vi "PixeLink MonitorAndSave_old.vi"(7 "Racine chemin de sauvegarde":path=path "G:/Développement de Programmes/Programmes/octo-labview/PixeLink - Homebrew/Data") -> ()   [LabVIEW 2014]
uses:
  <vilib>/addons/PixeLINK/Low Level Functions/ACQUISITION.llb/TDPU-Acquisition-StreamState.ctl
  <vilib>/addons/PixeLINK/Low Level Functions/CAMERA_FEATURES.llb/TDPU-CameraFeatures-FeatureIds.ctl
  <vilib>/addons/PixeLINK/Low Level Functions/CAMERA_FEATURES.llb/TDPU-CameraFeatures-FeatureFlags.ctl
panel:
  in  "Refresh Exposure":bool
  out "Div":dbl
  out "Imager Serial #":u32[](array[numeric])
  in  "Chemins de sauvegarde":path[](array[path])
  in  "Bind Path to Camera":bool
  in  "Automatic\nfolder naming":bool=TRUE
  in  "Imager":u32(ring)=741003962 items=["Cam 0"=95300230]
  out "Error OUT 2":errorcluster
  out "Error OUT":errorcluster
  in  "Overwrite?":bool
  in  "Snap current Data":bool
  in  "Save Data":bool
  out "Warning":bool
  out "Message":string
  in  "Indice":u32
  in  "Nom du fichier":string="tir"
  in  "Mode de Sauvegarde":u16(ring)=1 items=["Manuel", "Automatique"]
  out "Captured Image":dbl[][](graph)
  out "Waiting for Trigger":bool
  in  "Continuous Grab":bool
  in  "Snap Next frame":bool
  out "Camera Handle":u32
  in  "Stop Grab":bool
  in  "Trigger Type":enum16{"Free Running", "Software", "Hardware"}(ring)
  in  "Trigger Polarity":enum16{"Positive", "Negative"}(ring)
  in  "Refresh Trigger":bool
  in  "Exposure Time":dbl(slide) min=6.350000330712646e-05 max=10.0 scale=6.350000330712646e-05..10.0
  in  "stop":bool
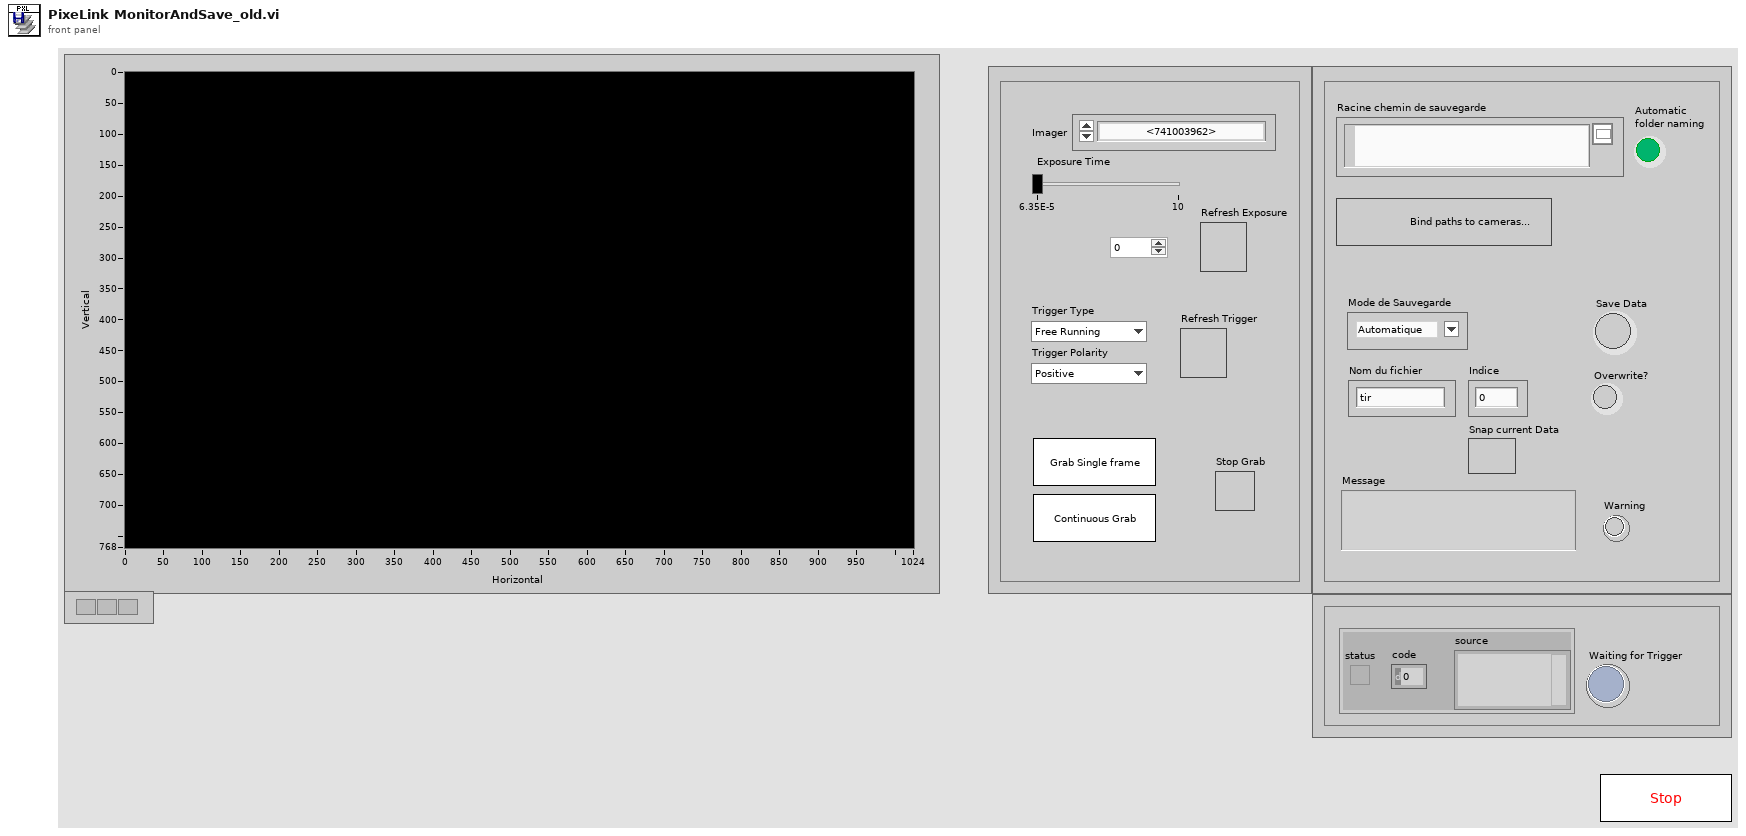
[diagram p1: front panel]
types:
  T1 = typedef "LVStringsAndValuesArrayTypeDef_U32.ctl" = cluster{"String":string, "Value":u32}[]
  T2 = typedef "TDPU-CameraFeatures-FeatureFlags.ctl" = u32
  T3 = typedef "TDPU-CameraFeatures-FeatureIds.ctl" = u32
  T4 = typedef "TDPU-Acquisition-StreamState.ctl" = u32
  T5 = typedef "TDPU-Identification-Camera_Info.ctl" = cluster{"VendorName":string, "ModelName":string, "Description":string, "SerialNumber":string, "FirmwareVersion":string, "FPGAVersion":string, "CameraName":string}
  T6 = typedef "TDPU-Acquisition-Frame_Desc.ctl" = cluster{"uSize":u32, "fFrameTime":dbl, "uFrameNumber":u32, "Brightness":cluster{"fValue":dbl}, "AutoExposure":cluster{"fValue":dbl}, "Sharpness":cluster{"fValue":dbl}, "WhiteBalance":cluster{"fValue":dbl}, "Hue":cluster{"fValue":dbl}, "Saturation":cluster{"fValue":dbl}, "Gamma":cluster{"fValue":dbl}, "Shutter":cluster{"fValue":dbl}, "Gain":cluster{"fValue":dbl}, "Iris":cluster{"fValue":dbl}, "Focus":cluster{"fValue":dbl}, "Temperature":cluster{"fValue":dbl}, "Trigger":cluster{"fMode":dbl, "fType":dbl, "fPolarity":dbl, "fDelay":dbl, "fParameter":dbl}, "Zoom":cluster{"fValue":dbl}, "Pan":cluster{"fValue":dbl}, "Tilt":cluster{"fValue":dbl}, "OpticalFilter":cluster{"fValue":dbl}, "GPIO":cluster{"fMode":dbl[], "fPolarity":dbl[], "fParameter1":dbl[], "fParameter2":dbl[], "fParameter3":dbl[]}, "FrameRate":cluster{"fValue":dbl}, "ROI":cluster{"fLeft":dbl, "fTop":dbl, "fWidth":dbl, "fHeight":dbl}, "Flip":cluster{"fHorizontal":dbl, "fVertical":dbl}, "PixelAddressingValue":cluster{"fValue":dbl}, "PixelFormat":cluster{"fValue":dbl}, "ExtendedShutter":cluster{"fKneePoint":dbl[]}, "AutoROI":cluster{"fLeft":dbl, "fTop":dbl, "fWidth":dbl, "fHeight":dbl}, "WhiteShading":cluster{"fRedGain":dbl, "fGreenGain":dbl, "fBlueGain":dbl}, "Rotate":cluster{"fValue":dbl}, "PixelAddressingMode":cluster{"fValue":dbl}}
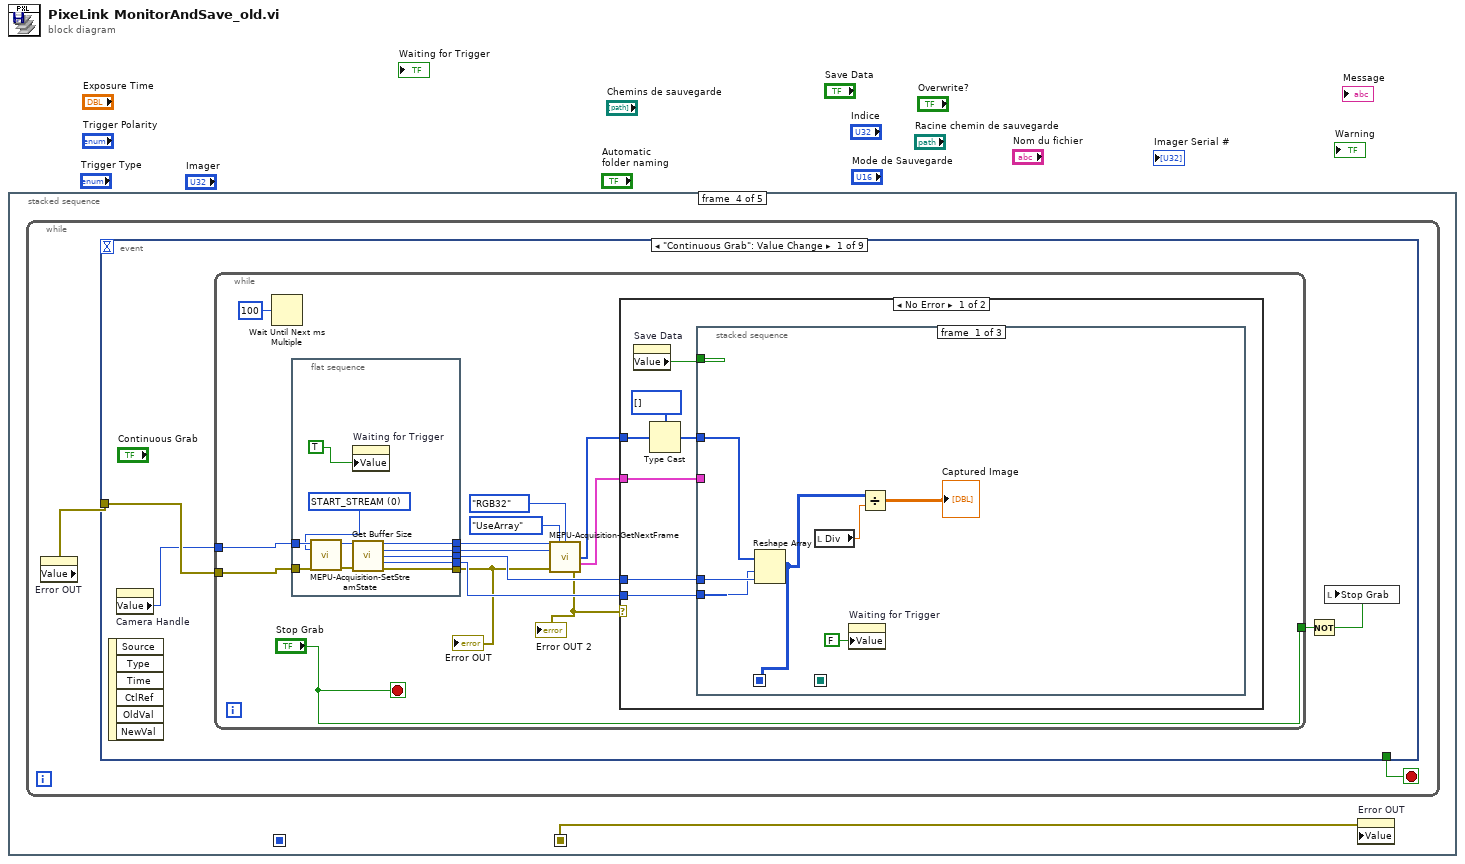
[diagram p0: block diagram]
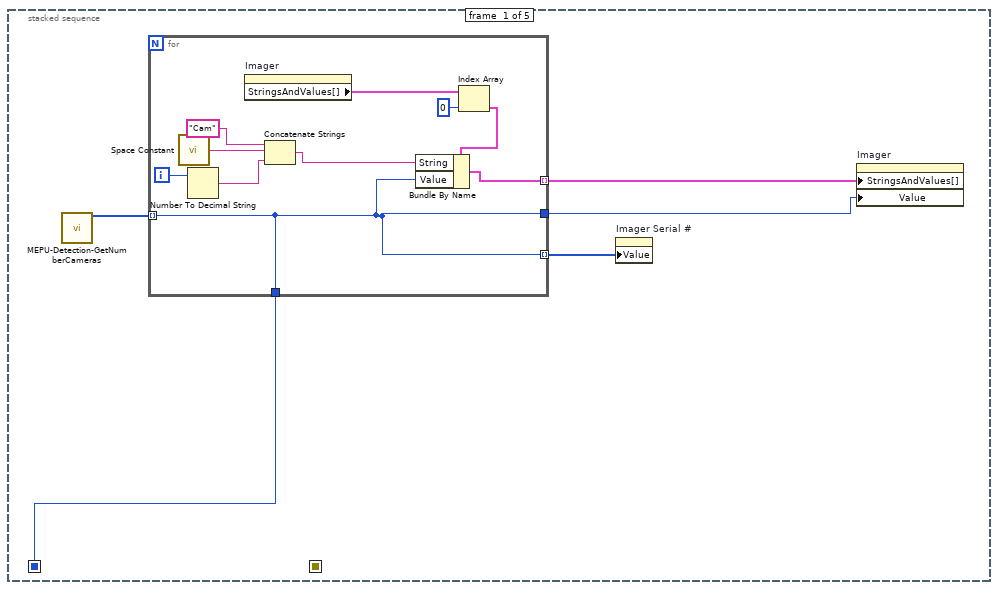
[diagram p2: hidden frame]
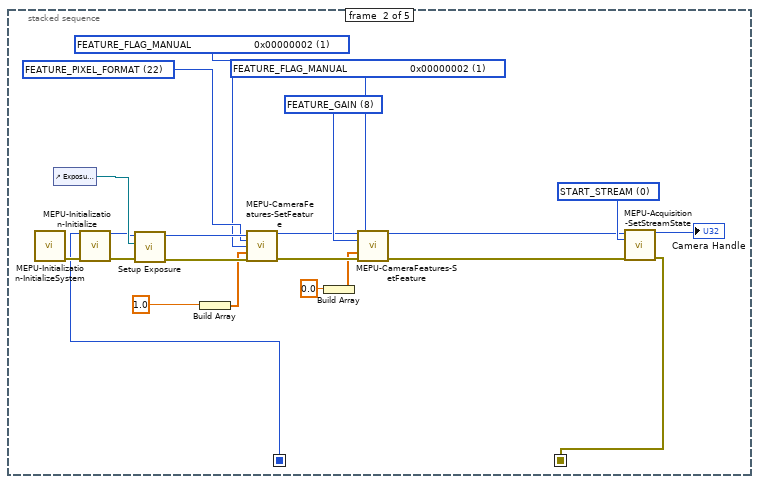
[diagram p3: hidden frame]
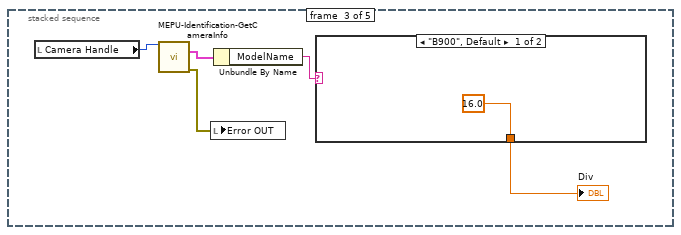
[diagram p4: hidden frame]
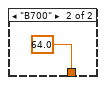
[diagram p5: hidden frame]
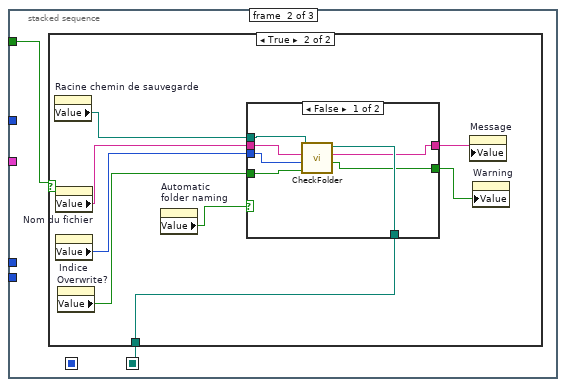
[diagram p6: hidden frame]
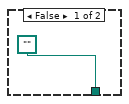
[diagram p7: hidden frame]
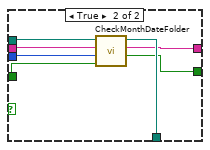
[diagram p8: hidden frame]
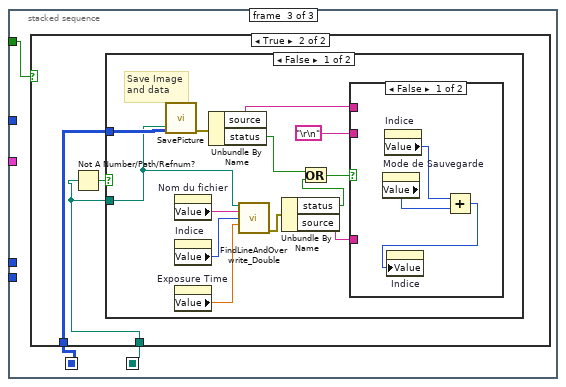
[diagram p9: hidden frame]
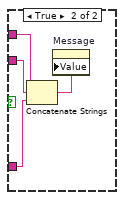
[diagram p11: hidden frame]
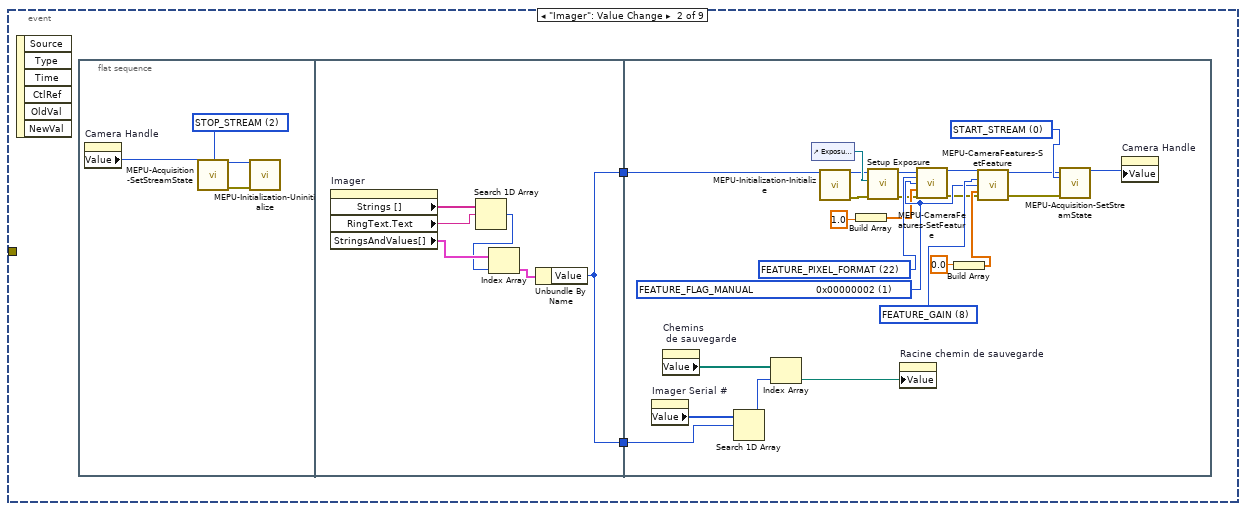
[diagram p14: hidden frame]
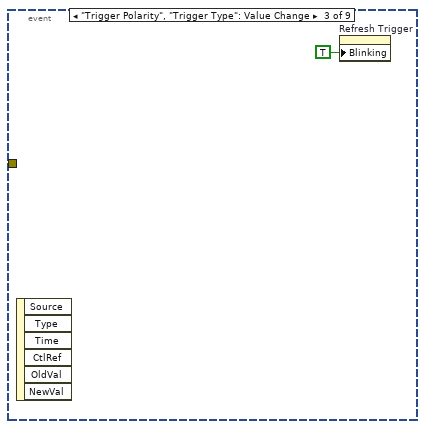
[diagram p15: hidden frame]
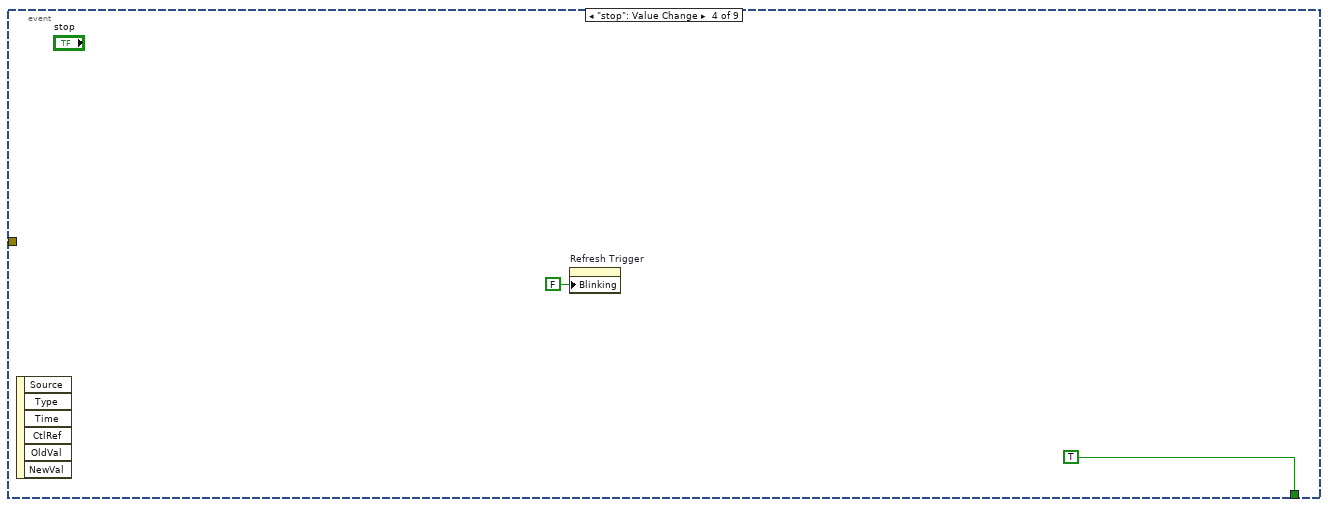
[diagram p16: hidden frame]
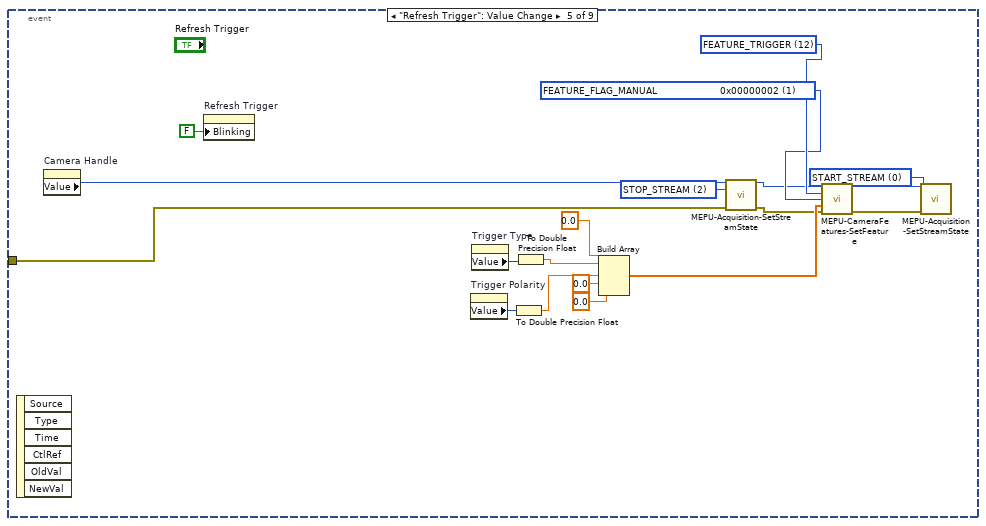
[diagram p17: hidden frame]
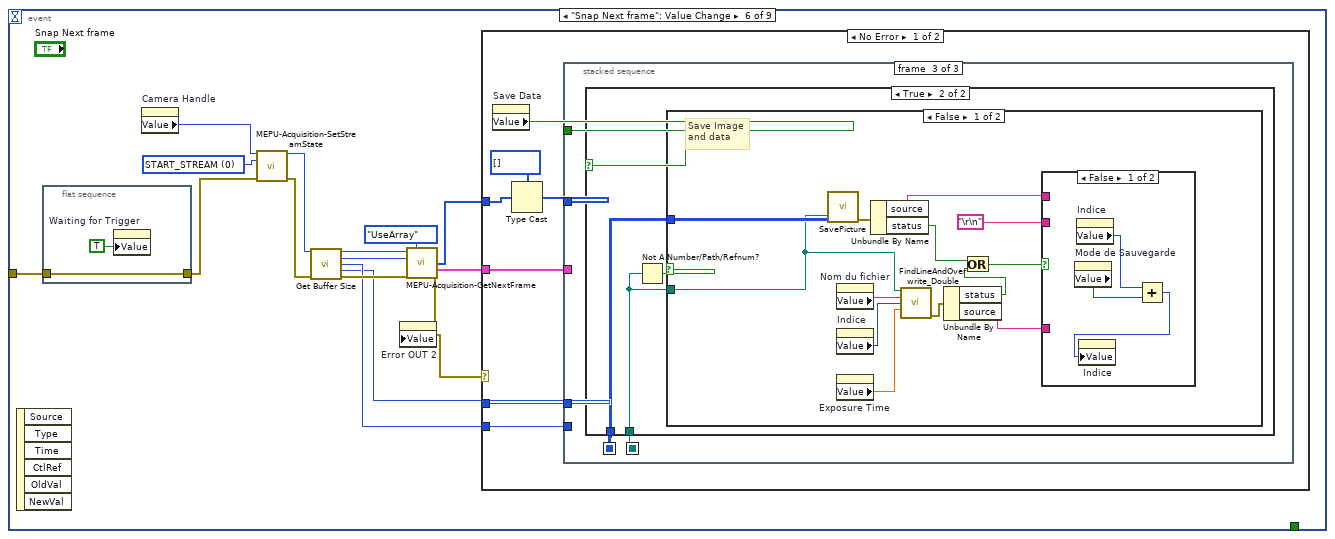
[diagram p18: hidden frame]
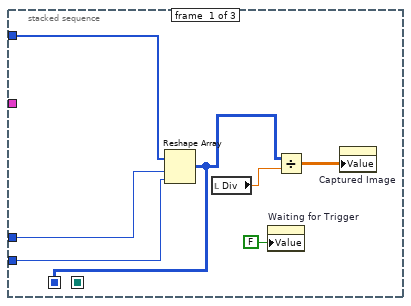
[diagram p19: hidden frame]
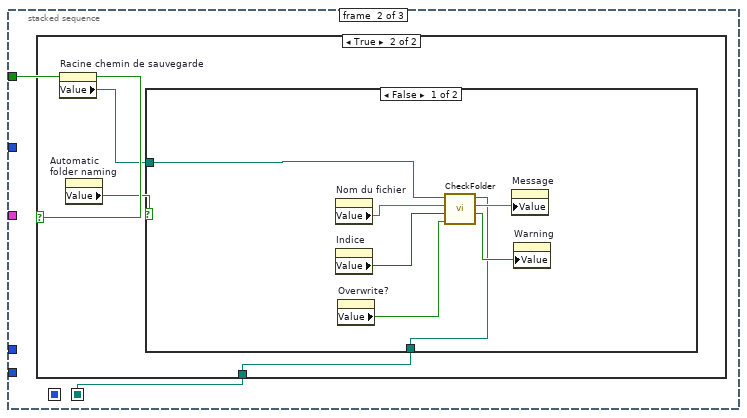
[diagram p20: hidden frame]
diagram:
  n1 = stacked-sequence {
    seq-local: [_ w26 _ _ _] -> [_ _ _ w45 _]
    seq-local: [w4 _ _ _ _] -> [_ w16 _ _ _]
    frame #0 {
      n2 = call <vilib>:"MEPU-Detection-GetNumberCameras.vi"() -> ("LV_SerialNumbers OUT"=w5:u32[])  [unwired: 13 in, 2 out]
      n3 = for {
        tunnel: w5 -> [w6] mode=indexing
        tunnel: [w10] -> w3 mode=indexing
        tunnel: [w6] -> w4
        tunnel: [w6] -> w2
        tunnel: [w6] -> w1 mode=indexing
        i -> [w15]
        n4 = call <vilib>:"Space Constant.vi"() -> ("String"=w13:string)
        n5 = Number To Decimal String(number=w15) -> (decimal integer string=w12:string)  [unwired: 1 in]
        n6 = property on="Imager" class="Ring (strict)"() -> ("StringsAndValues[]"=w9:T1)  [unwired: 2 in, 2 out]
        n7 = Concatenate Strings("Cam", w13, w12) -> (w11:string)
        n8 = Index Array(array=w9, index=0) -> (element=w7:cluster{"String":string, "Value":u32})
        n9 = Bundle By Name(cluster=w7, "String"=w11, "Value"=w6) -> (w10:cluster{"String":string, "Value":u32})
      }
      n10 = property on="Imager Serial #" class="Arr (strict)"("Value"=w1) -> ()  [unwired: 2 in, 2 out]
      n11 = property on="Imager" class="Ring (strict)"("StringsAndValues[]"=w3, "Value"=w2) -> ()  [unwired: 2 in, 2 out]
    }
    frame #1 {
      w21 = T2 1 items=["FEATURE_FLAG_PRESENCE                 0x00000001", "FEATURE_FLAG_MANUAL                     0x00000002", "FEATURE_FLAG_AUTO                         0x00000004", "FEATURE_FLAG_ONEPUSH                   0x00000008", "FEATURE_FLAG_OFF                            0x00000010", "FEATURE_FLAG_DESC_SUPPORTED    0x00000020", "FEATURE_FLAG_READ_ONLY               0x00000040"] ("uFlags IN")
      w20 = T3 8 items=["FEATURE_BRIGHTNESS", "FEATURE_EXPOSURE", "FEATURE_SHARPNESS", "FEATURE_WHITE_BAL", "FEATURE_HUE", "FEATURE_SATURATION", "FEATURE_GAMMA", "FEATURE_SHUTTER", "FEATURE_GAIN", "FEATURE_IRIS", "FEATURE_FOCUS", "FEATURE_TEMPERATURE", "FEATURE_TRIGGER", "FEATURE_ZOOM", "FEATURE_PAN", "FEATURE_TILT", "FEATURE_OPT_FILTER", "FEATURE_GPIO", "FEATURE_FRAME_RATE", "FEATURE_ROI", "FEATURE_FLIP", "FEATURE_PIXEL_ADDRESSING", "FEATURE_PIXEL_FORMAT", "FEATURE_EXTENDED_SHUTTER", "FEATURE_AUTO_ROI", "FEATURE_LOOKUP_TABLE", "FEATURE_MEMORY_CHANNEL", "FEATURE_WHITE_SHADING", "FEATURE_ROTATE", "FEATURE_IMAGER_CLK_DIVISOR", "FEATURE_TRIG_WITH_CNTRLD_LIGHT", "FEATURE_MAX_PIXEL_SIZE"] ("uFeatureId IN")
      w29 = T2 1 items=["FEATURE_FLAG_PRESENCE                 0x00000001", "FEATURE_FLAG_MANUAL                     0x00000002", "FEATURE_FLAG_AUTO                         0x00000004", "FEATURE_FLAG_ONEPUSH                   0x00000008", "FEATURE_FLAG_OFF                            0x00000010", "FEATURE_FLAG_DESC_SUPPORTED    0x00000020", "FEATURE_FLAG_READ_ONLY               0x00000040"] ("uFlags IN")
      w30 = T3 22 items=["FEATURE_BRIGHTNESS", "FEATURE_EXPOSURE", "FEATURE_SHARPNESS", "FEATURE_WHITE_BAL", "FEATURE_HUE", "FEATURE_SATURATION", "FEATURE_GAMMA", "FEATURE_SHUTTER", "FEATURE_GAIN", "FEATURE_IRIS", "FEATURE_FOCUS", "FEATURE_TEMPERATURE", "FEATURE_TRIGGER", "FEATURE_ZOOM", "FEATURE_PAN", "FEATURE_TILT", "FEATURE_OPT_FILTER", "FEATURE_GPIO", "FEATURE_FRAME_RATE", "FEATURE_ROI", "FEATURE_FLIP", "FEATURE_PIXEL_ADDRESSING", "FEATURE_PIXEL_FORMAT", "FEATURE_EXTENDED_SHUTTER", "FEATURE_AUTO_ROI", "FEATURE_LOOKUP_TABLE", "FEATURE_MEMORY_CHANNEL", "FEATURE_WHITE_SHADING", "FEATURE_ROTATE", "FEATURE_IMAGER_CLK_DIVISOR", "FEATURE_TRIG_WITH_CNTRLD_LIGHT", "FEATURE_MAX_PIXEL_SIZE"] ("uFeatureId IN")
      w36 = T4 0 items=["START_STREAM", "PAUSE_STREAM", "STOP_STREAM"] ("uStreamState IN")
      n12 = call <vilib>:"MEPU-Initialization-InitializeSystem.vi"() -> ("Error OUT"=w37:errorcluster)  [unwired: 15 in]
      n13 = control-ref of="Exposure Time"() -> (w35:refnum<vi>)
      n14 = call <vilib>:"MEPU-Initialization-Initialize.vi"("uSerialNumber IN"=w16, "Error IN"=w37) -> ("phCamera OUT"=w34:u32, "Error OUT"=w33:errorcluster)  [unwired: 11 in, 1 out]
      n15 = call "Setup Exposure.vi"("Error IN"=w33, "Shutter"=w35, "hCamera IN"=w34) -> ("Error OUT"=w32:errorcluster, "phCamera OUT"=w31:u32)  [unwired: 7 in]
      n16 = Build Array(1.0) -> (w27:dbl[])
      n17 = call <vilib>:"MEPU-CameraFeatures-SetFeature.vi"("hCamera IN"=w31, "uFeatureId IN"=w30, "uFlags IN"=w29, "pParms IN"=w27, "Error IN"=w32) -> ("hCamera OUT"=w19:u32, "Error OUT"=w24:errorcluster)  [unwired: 8 in, 1 out]
      n18 = Build Array(0.0) -> (w22:dbl[])
      n19 = call <vilib>:"MEPU-CameraFeatures-SetFeature.vi"("hCamera IN"=w19, "uFeatureId IN"=w20, "uFlags IN"=w21, "pParms IN"=w22, "Error IN"=w24) -> ("hCamera OUT"=w18:u32, "Error OUT"=w17:errorcluster)  [unwired: 8 in, 1 out]
      n20 = call <vilib>:"MEPU-Acquisition-SetStreamState.vi"("hCamera IN"=w18, "uStreamState IN"=w36, "Error IN"=w17) -> ("hCamera OUT"=→"Camera Handle":u32, "Error OUT"=w26:errorcluster)  [unwired: 11 in]
    }
    frame #2 {
      n21 = local read "Camera Handle"() -> (w42:u32)
      n22 = call <vilib>:"MEPU-Identification-GetCameraInfo.vi"("hCamera IN"=w42) -> ("pLVCameraInfo OUT"=w41:T5, "Error OUT"=w38:errorcluster)  [unwired: 12 in, 1 out]
      n23 = local write "Error OUT"(w38) -> ()
      n24 = Unbundle By Name(w41) -> ("ModelName"=w40:string)
      n25 = case shown="\"B900\", Default" w40 {
        tunnel: [16.0 64.0] -> w39
        frame "B900", Default {
        }
        frame "B700" {
        }
      }
      "Div" <- w39
    }
    frame #3 {
      n26 = while {
        stop <- w47 stop-if-true
        n27 = property on="Error OUT" class="Clust (strict)"() -> ("Value"=w46:errorcluster)  [unwired: 2 in, 2 out]
        n28 = event shown="[0] \"Continuous Grab\": Value Change" {
          selector: _ -> [_ _ _ _ _ _ _ _ _]
          dyn-events: _ -> [_ _ _ _ _ _ _ _ _]
          timeout: _ -> [_ _ _ _ _ _ _ _ _]
          tunnel: w46 -> [w51 _ _ _ w189 w207 _ _ _]
          tunnel: [_ _ _ TRUE _ _ _ _ _] -> w47
          event "Continuous Grab": Value Change {
            n29 = event-data() -> ()  [unwired: 1 in, 6 out]
            n30 = property on="Camera Handle" class="DigNum (strict)"() -> ("Value"=w50:u32)  [unwired: 2 in, 2 out]
            n31 = while {
              tunnel: w50 -> [w65]
              tunnel: w51 -> [w59]
              tunnel: ["Stop Grab"] -> w49
              stop <- "Stop Grab" stop-if-true
              n32 = Wait Until Next ms Multiple(millisecond multiple=u32 100) -> ()  [unwired: 1 out]
              n33 = flat-sequence {
                tunnel: w65 -> [w132]
                tunnel: [w141] -> w64
                tunnel: [w140] -> w63
                tunnel: [w139] -> w56
                tunnel: w59 -> [w135]
                tunnel: [w138] -> w58
                tunnel: [w137] -> w57
                frame #0 {
                  w131 = T4 0 items=["START_STREAM", "PAUSE_STREAM", "STOP_STREAM"] ("uStreamState IN")
                  n34 = call <vilib>:"MEPU-Acquisition-SetStreamState.vi"("hCamera IN"=w132, "uStreamState IN"=w131, "Error IN"=w135) -> ("hCamera OUT"=w133:u32, "Error OUT"=w134:errorcluster)  [unwired: 11 in]
                  n35 = property on="Waiting for Trigger" class="Bool (strict)"("Value"=TRUE ("Waiting for Trigger")) -> ()  [unwired: 2 in, 2 out]
                  n36 = call "Get Buffer Size.vi"("phCamera IN"=w133, "Error IN"=w134) -> ("phCamera OUT"=w141:u32, "uBufferSize OUT"=w140:u32, "uWidth OUT"=w138:u32, "uHeight OUT"=w137:u32, "Error OUT"=w139:errorcluster)  [unwired: 8 in, 1 out]
                }
              }
              n37 = call <vilib>:"MEPU-Acquisition-GetNextFrame.vi"("hCamera IN"=w64, "Mode IN"=enum16{"UseArray", "UsePointer"}."UseArray", "OutputMode IN"=enum16{"Default", "RGB24", "RGB32"}."RGB32", "uBufferSize IN"=w63, "Error IN"=w56) -> ("Data OUT"=w60:u8[], "pDescriptor"=w54:T6, "Error OUT"=w55:errorcluster)  [unwired: 6 in, 2 out]
              "Error OUT 2" <- w55
              n38 = case shown="No Error" w55 {
                tunnel: w60 -> [w72 _]
                tunnel: w58 -> [w69 _]
                tunnel: w57 -> [w68 _]
                tunnel: w54 -> [w66 _]
                frame No Error {
                  n39 = property on="Save Data" class="Bool (strict)"() -> ("Value"=w67:bool)  [unwired: 2 in, 2 out]
                  n40 = Type Cast(type=u16[] [] ("Data OUT"), x=w72) -> (*(type *) &x=w70:u16[])
                  n41 = stacked-sequence {
                    seq-local: [_ w81 _] -> [_ _ w107]
                    seq-local: [w75 _ _] -> [_ _ w105]
                    tunnel: w70 -> [w79 _ _]
                    tunnel: w69 -> [w78 _ _]
                    tunnel: w68 -> [w77 _ _]
                    tunnel: w67 -> [_ w80 w106]
                    tunnel: w66 -> [_ _ _]
                    frame #0 {
                      n42 = Reshape Array(w79, w77, w78) -> (w75:u16[][])
                      n43 = local read "Div"() -> (w74:dbl)
                      n44 = property on="Waiting for Trigger" class="Bool (strict)"("Value"=FALSE ("Waiting for Trigger")) -> ()  [unwired: 2 in, 2 out]
                      n45 = Divide(x=w75, y=w74) -> (x/y=→"Captured Image":dbl[][])
                    }
                    frame #1 {
                      n46 = case shown="True" w80 {
                        tunnel: [path "" ("File Path") w86] -> w81
                        frame False {
                        }
                        frame True {
                          n47 = property on="Racine chemin de sauvegarde" class="Path"() -> ("Value"=w87:path)  [unwired: 2 in, 2 out]
                          n48 = property on="Nom du fichier" class="Str"() -> ("Value"=w88:string)  [unwired: 2 in, 2 out]
                          n49 = property on="Indice" class="DigNum (strict)"() -> ("Value"=w89:u32)  [unwired: 2 in, 2 out]
                          n50 = property on="Overwrite?" class="Bool (strict)"() -> ("Value"=w90:bool)  [unwired: 2 in, 2 out]
                          n51 = property on="Automatic\nfolder naming" class="Bool (strict)"() -> ("Value"=w83:bool)  [unwired: 2 in, 2 out]
                          n52 = case shown="False" w83 {
                            tunnel: w90 -> [w95 w104]
                            tunnel: w89 -> [w96 w103]
                            tunnel: w88 -> [w97 w102]
                            tunnel: w87 -> [w94 w101]
                            tunnel: [w93 w100] -> w86
                            tunnel: [w92 w99] -> w85
                            tunnel: [w91 w98] -> w84
                            frame False {
                              n53 = call "CheckFolder.vi"("Overwrite?"=w95, "Index"=w96, "File Name"=w97, "Folder Path Control"=w94) -> ("Warning"=w91:bool, "Message"=w92:string, "File Path"=w93:path)  [unwired: 5 in]
                            }
                            frame True {
                              n54 = call "CheckMonthDateFolder.vi"("Overwrite?"=w104, "Index"=w103, "File Name"=w102, "Folder Path Control"=w101) -> ("Warning"=w98:bool, "Message"=w99:string, "File Path"=w100:path)  [unwired: 5 in]
                            }
                          }
                          n55 = property on="Message" class="Str"("Value"=w85) -> ()  [unwired: 2 in, 2 out]
                          n56 = property on="Warning" class="Bool (strict)"("Value"=w84) -> ()  [unwired: 2 in, 2 out]
                        }
                      }
                    }
                    frame #2 {
                      n57 = case shown="True" w106 {
                        tunnel: w107 -> [_ w109]
                        tunnel: w105 -> [_ w108]
                        frame False {
                        }
                        frame True {
                          n58 = Not A Number/Path/Refnum?(number/path/refnum=w109) -> (NaN/Path/Refnum?=w110:bool)
                          n59 = case shown="False" w110 {
                            tunnel: w109 -> [w114 _]
                            tunnel: w108 -> [w116 _]
                            frame False {
                              # "Save Image\nand data"
                              n60 = call "SavePicture.vi"("File Path"=w114, "Image Pixels (U16)"=w116) -> ("error out"=w122:errorcluster)  [unwired: 9 in]
                              n61 = property on="Nom du fichier" class="Str"() -> ("Value"=w113:string)  [unwired: 2 in, 2 out]
                              n62 = property on="Indice" class="DigNum (strict)"() -> ("Value"=w112:u32)  [unwired: 2 in, 2 out]
                              n63 = property on="Exposure Time" class="Slide (strict)"() -> ("Value"=w111:dbl)  [unwired: 2 in, 2 out]
                              n64 = Unbundle By Name(w122) -> ("source"=w119:string, "status"=w120:bool)
                              n65 = call "FindLineAndOverwrite_Double.vi"("Exposure path"=w114, "Name"=w113, "Index"=w112, "Exposure"=w111) -> ("error out"=w115:errorcluster)  [unwired: 11 in]
                              n66 = Unbundle By Name(w115) -> ("status"=w121:bool, "source"=w123:string)
                              n67 = Or(x=w120, y=w121) -> (x .or. y?=w118:bool)
                              n68 = case shown="False" w118 {
                                tunnel: w123 -> [_ w127]
                                tunnel: w119 -> [_ w130]
                                tunnel: "\r\n" -> [_ w128]
                                frame False {
                                n69 = property on="Mode de Sauvegarde" class="Ring (strict)"() -> ("Value"=w125:u16)  [unwired: 2 in, 2 out]
                                n70 = property on="Indice" class="DigNum (strict)"() -> ("Value"=w126:u32)  [unwired: 2 in, 2 out]
                                n71 = Add(x=w126, y=w125) -> (x+y=w124:u32)
                                n72 = property on="Indice" class="DigNum (strict)"("Value"=w124) -> ()  [unwired: 2 in, 2 out]
                                }
                                frame True {
                                n73 = Concatenate Strings(w130, w128, w127) -> (w129:string)
                                n74 = property on="Message" class="Str"("Value"=w129) -> ()  [unwired: 2 in, 2 out]
                                }
                              }
                            }
                            frame True {
                            }
                          }
                        }
                      }
                    }
                  }
                }
                frame Error {
                }
              }
              "Error OUT" <- w56
            }
            n75 = Not(x=w49) -> (.not. x?=w48:bool)
            n76 = local write "Stop Grab"(w48) -> ()
          }
          event "Imager": Value Change {
            n77 = event-data() -> ()  [unwired: 1 in, 6 out]
            n78 = flat-sequence {
              tunnel: [w148] -> w143
              tunnel: [w148] -> w142
              tunnel: w143 -> [w159]
              tunnel: w142 -> [w155]
              frame #0 {
                w145 = T4 2 items=["START_STREAM", "PAUSE_STREAM", "STOP_STREAM"] ("uStreamState IN")
                n79 = property on="Camera Handle" class="DigNum (strict)"() -> ("Value"=w144:u32)  [unwired: 2 in, 2 out]
                n80 = call <vilib>:"MEPU-Acquisition-SetStreamState.vi"("hCamera IN"=w144, "uStreamState IN"=w145) -> ("hCamera OUT"=w146:u32, "Error OUT"=w147:errorcluster)  [unwired: 12 in]
                n81 = call <vilib>:"MEPU-Initialization-Uninitialize.vi"("hCamera IN"=w146, "Error IN"=w147) -> ()  [unwired: 13 in, 1 out]
              }
              frame #1 {
                n82 = property on="Imager" class="Ring (strict)"() -> ("Strings []"=w153:string[], "RingText.Text"=w152:string, "StringsAndValues[]"=w151:T1)  [unwired: 2 in, 2 out]
                n83 = Search 1D Array(1D array=w153, element=w152) -> (index of element=w150:i32)  [unwired: 1 in]
                n84 = Index Array(array=w151, index=w150) -> (element=w149:cluster{"String":string, "Value":u32})
                n85 = Unbundle By Name(w149) -> ("Value"=w148:u32)
              }
              frame #2 {
                w176 = T4 0 items=["START_STREAM", "PAUSE_STREAM", "STOP_STREAM"] ("uStreamState IN")
                w173 = T3 8 items=["FEATURE_BRIGHTNESS", "FEATURE_EXPOSURE", "FEATURE_SHARPNESS", "FEATURE_WHITE_BAL", "FEATURE_HUE", "FEATURE_SATURATION", "FEATURE_GAMMA", "FEATURE_SHUTTER", "FEATURE_GAIN", "FEATURE_IRIS", "FEATURE_FOCUS", "FEATURE_TEMPERATURE", "FEATURE_TRIGGER", "FEATURE_ZOOM", "FEATURE_PAN", "FEATURE_TILT", "FEATURE_OPT_FILTER", "FEATURE_GPIO", "FEATURE_FRAME_RATE", "FEATURE_ROI", "FEATURE_FLIP", "FEATURE_PIXEL_ADDRESSING", "FEATURE_PIXEL_FORMAT", "FEATURE_EXTENDED_SHUTTER", "FEATURE_AUTO_ROI", "FEATURE_LOOKUP_TABLE", "FEATURE_MEMORY_CHANNEL", "FEATURE_WHITE_SHADING", "FEATURE_ROTATE", "FEATURE_IMAGER_CLK_DIVISOR", "FEATURE_TRIG_WITH_CNTRLD_LIGHT", "FEATURE_MAX_PIXEL_SIZE"] ("uFeatureId IN")
                w172 = T2 1 items=["FEATURE_FLAG_PRESENCE                 0x00000001", "FEATURE_FLAG_MANUAL                     0x00000002", "FEATURE_FLAG_AUTO                         0x00000004", "FEATURE_FLAG_ONEPUSH                   0x00000008", "FEATURE_FLAG_OFF                            0x00000010", "FEATURE_FLAG_DESC_SUPPORTED    0x00000020", "FEATURE_FLAG_READ_ONLY               0x00000040"] ("uFlags IN")
                w167 = T3 22 items=["FEATURE_BRIGHTNESS", "FEATURE_EXPOSURE", "FEATURE_SHARPNESS", "FEATURE_WHITE_BAL", "FEATURE_HUE", "FEATURE_SATURATION", "FEATURE_GAMMA", "FEATURE_SHUTTER", "FEATURE_GAIN", "FEATURE_IRIS", "FEATURE_FOCUS", "FEATURE_TEMPERATURE", "FEATURE_TRIGGER", "FEATURE_ZOOM", "FEATURE_PAN", "FEATURE_TILT", "FEATURE_OPT_FILTER", "FEATURE_GPIO", "FEATURE_FRAME_RATE", "FEATURE_ROI", "FEATURE_FLIP", "FEATURE_PIXEL_ADDRESSING", "FEATURE_PIXEL_FORMAT", "FEATURE_EXTENDED_SHUTTER", "FEATURE_AUTO_ROI", "FEATURE_LOOKUP_TABLE", "FEATURE_MEMORY_CHANNEL", "FEATURE_WHITE_SHADING", "FEATURE_ROTATE", "FEATURE_IMAGER_CLK_DIVISOR", "FEATURE_TRIG_WITH_CNTRLD_LIGHT", "FEATURE_MAX_PIXEL_SIZE"] ("uFeatureId IN")
                n86 = property on="Imager Serial #" class="Arr (strict)"() -> ("Value"=w156:u32[])  [unwired: 2 in, 2 out]
                n87 = property on="Chemins\n de sauvegarde" class="Arr (strict)"() -> ("Value"=w158:path[])  [unwired: 2 in, 2 out]
                n88 = Search 1D Array(1D array=w156, element=w155) -> (index of element=w154:i32)  [unwired: 1 in]
                n89 = Index Array(array=w158, index=w154) -> (element=w157:path)
                n90 = control-ref of="Exposure Time"() -> (w162:refnum<vi>)
                n91 = call <vilib>:"MEPU-Initialization-Initialize.vi"("uSerialNumber IN"=w159) -> ("phCamera OUT"=w161:u32, "Error OUT"=w160:errorcluster)  [unwired: 12 in, 1 out]
                n92 = Build Array(1.0) -> (w166:dbl[])
                n93 = call "Setup Exposure.vi"("Error IN"=w160, "Shutter"=w162, "hCamera IN"=w161) -> ("Error OUT"=w164:errorcluster, "phCamera OUT"=w163:u32)  [unwired: 7 in]
                n94 = property on="Racine chemin de sauvegarde" class="Path"("Value"=w157) -> ()  [unwired: 2 in, 2 out]
                n95 = call <vilib>:"MEPU-CameraFeatures-SetFeature.vi"("hCamera IN"=w163, "uFeatureId IN"=w167, "uFlags IN"=w172, "pParms IN"=w166, "Error IN"=w164) -> ("hCamera OUT"=w168:u32, "Error OUT"=w169:errorcluster)  [unwired: 8 in, 1 out]
                n96 = Build Array(0.0) -> (w171:dbl[])
                n97 = call <vilib>:"MEPU-CameraFeatures-SetFeature.vi"("hCamera IN"=w168, "uFeatureId IN"=w173, "uFlags IN"=w172, "pParms IN"=w171, "Error IN"=w169) -> ("hCamera OUT"=w174:u32, "Error OUT"=w175:errorcluster)  [unwired: 8 in, 1 out]
                n98 = call <vilib>:"MEPU-Acquisition-SetStreamState.vi"("hCamera IN"=w174, "uStreamState IN"=w176, "Error IN"=w175) -> ("hCamera OUT"=w177:u32)  [unwired: 11 in, 1 out]
                n99 = property on="Camera Handle" class="DigNum (strict)"("Value"=w177) -> ()  [unwired: 2 in, 2 out]
              }
            }
          }
          event "Trigger Polarity", "Trigger Type": Value Change {
            n100 = event-data() -> ()  [unwired: 1 in, 6 out]
            n101 = property on="Refresh Trigger" class="Bool"("Blinking"=TRUE) -> ()  [unwired: 2 in, 2 out]
          }
          event "stop": Value Change {
            n102 = event-data() -> ()  [unwired: 1 in, 6 out]
            n103 = property on="Refresh Trigger" class="Bool"("Blinking"=FALSE) -> ()  [unwired: 2 in, 2 out]
          }
          event "Refresh Trigger": Value Change {
            w183 = T4 2 items=["START_STREAM", "PAUSE_STREAM", "STOP_STREAM"] ("uStreamState IN")
            w184 = T4 0 items=["START_STREAM", "PAUSE_STREAM", "STOP_STREAM"] ("uStreamState IN")
            w198 = T2 1 items=["FEATURE_FLAG_PRESENCE                 0x00000001", "FEATURE_FLAG_MANUAL                     0x00000002", "FEATURE_FLAG_AUTO                         0x00000004", "FEATURE_FLAG_ONEPUSH                   0x00000008", "FEATURE_FLAG_OFF                            0x00000010", "FEATURE_FLAG_DESC_SUPPORTED    0x00000020", "FEATURE_FLAG_READ_ONLY               0x00000040"] ("uFlags IN")
            w199 = T3 12 items=["FEATURE_BRIGHTNESS", "FEATURE_EXPOSURE", "FEATURE_SHARPNESS", "FEATURE_WHITE_BAL", "FEATURE_HUE", "FEATURE_SATURATION", "FEATURE_GAMMA", "FEATURE_SHUTTER", "FEATURE_GAIN", "FEATURE_IRIS", "FEATURE_FOCUS", "FEATURE_TEMPERATURE", "FEATURE_TRIGGER", "FEATURE_ZOOM", "FEATURE_PAN", "FEATURE_TILT", "FEATURE_OPT_FILTER", "FEATURE_GPIO", "FEATURE_FRAME_RATE", "FEATURE_ROI", "FEATURE_FLIP", "FEATURE_PIXEL_ADDRESSING", "FEATURE_PIXEL_FORMAT", "FEATURE_EXTENDED_SHUTTER", "FEATURE_AUTO_ROI", "FEATURE_LOOKUP_TABLE", "FEATURE_MEMORY_CHANNEL", "FEATURE_WHITE_SHADING", "FEATURE_ROTATE", "FEATURE_IMAGER_CLK_DIVISOR", "FEATURE_TRIG_WITH_CNTRLD_LIGHT", "FEATURE_MAX_PIXEL_SIZE"] ("uFeatureId IN")
            n104 = event-data() -> ()  [unwired: 1 in, 6 out]
            n105 = property on="Camera Handle" class="DigNum (strict)"() -> ("Value"=w181:u32)  [unwired: 2 in, 2 out]
            n106 = property on="Refresh Trigger" class="Bool"("Blinking"=FALSE) -> ()  [unwired: 2 in, 2 out]
            n107 = property on="Trigger Polarity" class="Enum (strict)"() -> ("Value"=w194:enum16{"Positive", "Negative"})  [unwired: 2 in, 2 out]
            n108 = property on="Trigger Type" class="Enum (strict)"() -> ("Value"=w196:enum16{"Free Running", "Software", "Hardware"})  [unwired: 2 in, 2 out]
            n109 = To Double Precision Float(number=w194) -> (double precision float=w193:dbl)
            n110 = To Double Precision Float(number=w196) -> (double precision float=w195:dbl)
            n111 = Build Array(0.0 ("element"), w195, w193, 0.0 ("element"), 0.0 ("element")) -> (w190:dbl[])
            n112 = call <vilib>:"MEPU-Acquisition-SetStreamState.vi"("hCamera IN"=w181, "uStreamState IN"=w183, "Error IN"=w189) -> ("hCamera OUT"=w188:u32, "Error OUT"=w187:errorcluster)  [unwired: 11 in]
            n113 = call <vilib>:"MEPU-CameraFeatures-SetFeature.vi"("hCamera IN"=w188, "uFeatureId IN"=w199, "uFlags IN"=w198, "pParms IN"=w190, "Error IN"=w187) -> ("hCamera OUT"=w185:u32, "Error OUT"=w186:errorcluster)  [unwired: 9 out]
            n114 = call <vilib>:"MEPU-Acquisition-SetStreamState.vi"("hCamera IN"=w185, "uStreamState IN"=w184, "Error IN"=w186) -> ()  [unwired: 11 in, 2 out]
          }
          event "Snap Next frame": Value Change {
            w210 = T4 0 items=["START_STREAM", "PAUSE_STREAM", "STOP_STREAM"] ("uStreamState IN")
            n115 = event-data() -> ()  [unwired: 1 in, 6 out]
            n116 = flat-sequence {
              tunnel: w207 -> [w275]
              tunnel: [w275] -> w206
              frame #0 {
                n117 = property on="Waiting for Trigger" class="Bool (strict)"("Value"=TRUE ("Waiting for Trigger")) -> ()  [unwired: 2 in, 2 out]
              }
            }
            n118 = property on="Camera Handle" class="DigNum (strict)"() -> ("Value"=w200:u32)  [unwired: 2 in, 2 out]
            n119 = call <vilib>:"MEPU-Acquisition-SetStreamState.vi"("hCamera IN"=w200, "uStreamState IN"=w210, "Error IN"=w206) -> ("hCamera OUT"=w209:u32, "Error OUT"=w208:errorcluster)  [unwired: 11 in]
            n120 = call "Get Buffer Size.vi"("phCamera IN"=w209, "Error IN"=w208) -> ("phCamera OUT"=w214:u32, "uBufferSize OUT"=w212:u32, "uWidth OUT"=w203:u32, "uHeight OUT"=w202:u32, "Error OUT"=w213:errorcluster)  [unwired: 8 in, 1 out]
            n121 = call <vilib>:"MEPU-Acquisition-GetNextFrame.vi"("hCamera IN"=w214, "Mode IN"=enum16{"UseArray", "UsePointer"}."UseArray", "uBufferSize IN"=w212, "Error IN"=w213) -> ("Data OUT"=w205:u8[], "pDescriptor"=w201:T6, "Error OUT"=w204:errorcluster)  [unwired: 7 in, 2 out]
            n122 = property on="Error OUT 2" class="Clust (strict)"("Value"=w204) -> ()  [unwired: 2 in, 2 out]
            n123 = case shown="No Error" w204 {
              tunnel: w205 -> [w218 _]
              tunnel: w203 -> [w217 _]
              tunnel: w202 -> [w216 _]
              tunnel: w201 -> [w215 _]
              frame No Error {
                n124 = property on="Save Data" class="Bool (strict)"() -> ("Value"=w219:bool)  [unwired: 2 in, 2 out]
                n125 = Type Cast(type=u16[] [] ("Data OUT"), x=w218) -> (*(type *) &x=w220:u16[])
                n126 = stacked-sequence {
                  seq-local: [_ w230 _] -> [_ _ w251]
                  seq-local: [w223 _ _] -> [_ _ w249]
                  tunnel: w220 -> [w228 _ _]
                  tunnel: w219 -> [_ w229 w250]
                  tunnel: w217 -> [w226 _ _]
                  tunnel: w216 -> [w225 _ _]
                  tunnel: w215 -> [_ _ _]
                  frame #0 {
                    n127 = Reshape Array(w228, w225, w226) -> (w223:u16[][])
                    n128 = local read "Div"() -> (w224:dbl)
                    n129 = property on="Waiting for Trigger" class="Bool (strict)"("Value"=FALSE ("Waiting for Trigger")) -> ()  [unwired: 2 in, 2 out]
                    n130 = Divide(x=w223, y=w224) -> (x/y=w222:dbl[][])
                    n131 = property on="Captured Image" class="IntGraph (strict)"("Value"=w222) -> ()  [unwired: 2 in, 2 out]
                  }
                  frame #1 {
                    n132 = case shown="True" w229 {
                      tunnel: [path "" ("File Path") w234] -> w230
                      frame False {
                      }
                      frame True {
                        n133 = property on="Racine chemin de sauvegarde" class="Path"() -> ("Value"=w232:path)  [unwired: 2 in, 2 out]
                        n134 = property on="Automatic\nfolder naming" class="Bool (strict)"() -> ("Value"=w233:bool)  [unwired: 2 in, 2 out]
                        n135 = case shown="False" w233 {
                          tunnel: [w235 w242] -> w234
                          tunnel: w232 -> [w241 w243]
                          frame False {
                            n136 = property on="Nom du fichier" class="Str"() -> ("Value"=w238:string)  [unwired: 2 in, 2 out]
                            n137 = property on="Indice" class="DigNum (strict)"() -> ("Value"=w237:u32)  [unwired: 2 in, 2 out]
                            n138 = property on="Overwrite?" class="Bool (strict)"() -> ("Value"=w236:bool)  [unwired: 2 in, 2 out]
                            n139 = call "CheckFolder.vi"("Overwrite?"=w236, "Index"=w237, "File Name"=w238, "Folder Path Control"=w241) -> ("Warning"=w239:bool, "Message"=w240:string, "File Path"=w235:path)  [unwired: 5 in]
                            n140 = property on="Message" class="Str"("Value"=w240) -> ()  [unwired: 2 in, 2 out]
                            n141 = property on="Warning" class="Bool (strict)"("Value"=w239) -> ()  [unwired: 2 in, 2 out]
                          }
                          frame True {
                            n142 = property on="Nom du fichier" class="Str"() -> ("Value"=w246:string)  [unwired: 2 in, 2 out]
                            n143 = property on="Indice" class="DigNum (strict)"() -> ("Value"=w247:u32)  [unwired: 2 in, 2 out]
                            n144 = property on="Overwrite?" class="Bool (strict)"() -> ("Value"=w248:bool)  [unwired: 2 in, 2 out]
                            n145 = call "CheckMonthDateFolder.vi"("Overwrite?"=w248, "Index"=w247, "File Name"=w246, "Folder Path Control"=w243) -> ("Warning"=w244:bool, "Message"=w245:string, "File Path"=w242:path)  [unwired: 5 in]
                            n146 = property on="Warning" class="Bool (strict)"("Value"=w244) -> ()  [unwired: 2 in, 2 out]
                            n147 = property on="Message" class="Str"("Value"=w245) -> ()  [unwired: 2 in, 2 out]
                          }
                        }
                      }
                    }
                  }
                  frame #2 {
                    n148 = case shown="True" w250 {
                      tunnel: w251 -> [_ w253]
                      tunnel: w249 -> [_ w252]
                      frame False {
                      }
                      frame True {
                        n149 = Not A Number/Path/Refnum?(number/path/refnum=w253) -> (NaN/Path/Refnum?=w254:bool)
                        n150 = case shown="False" w254 {
                          tunnel: w253 -> [w258 _]
                          tunnel: w252 -> [w260 _]
                          frame False {
                            # "Save Image\nand data"
                            n151 = call "SavePicture.vi"("File Path"=w258, "Image Pixels (U16)"=w260) -> ("error out"=w266:errorcluster)  [unwired: 9 in]
                            n152 = property on="Nom du fichier" class="Str"() -> ("Value"=w257:string)  [unwired: 2 in, 2 out]
                            n153 = property on="Indice" class="DigNum (strict)"() -> ("Value"=w256:u32)  [unwired: 2 in, 2 out]
                            n154 = property on="Exposure Time" class="Slide (strict)"() -> ("Value"=w255:dbl)  [unwired: 2 in, 2 out]
                            n155 = Unbundle By Name(w266) -> ("source"=w263:string, "status"=w264:bool)
                            n156 = call "FindLineAndOverwrite_Double.vi"("Exposure path"=w258, "Name"=w257, "Index"=w256, "Exposure"=w255) -> ("error out"=w259:errorcluster)  [unwired: 11 in]
                            n157 = Unbundle By Name(w259) -> ("status"=w265:bool, "source"=w267:string)
                            n158 = Or(x=w264, y=w265) -> (x .or. y?=w262:bool)
                            n159 = case shown="False" w262 {
                              tunnel: w267 -> [_ w271]
                              tunnel: w263 -> [_ w274]
                              tunnel: "\r\n" -> [_ w272]
                              frame False {
                                n160 = property on="Mode de Sauvegarde" class="Ring (strict)"() -> ("Value"=w269:u16)  [unwired: 2 in, 2 out]
                                n161 = property on="Indice" class="DigNum (strict)"() -> ("Value"=w270:u32)  [unwired: 2 in, 2 out]
                                n162 = Add(x=w270, y=w269) -> (x+y=w268:u32)
                                n163 = property on="Indice" class="DigNum (strict)"("Value"=w268) -> ()  [unwired: 2 in, 2 out]
                              }
                              frame True {
                                n164 = Concatenate Strings(w274, w272, w271) -> (w273:string)
                                n165 = property on="Message" class="Str"("Value"=w273) -> ()  [unwired: 2 in, 2 out]
                              }
                            }
                          }
                          frame True {
                          }
                        }
                      }
                    }
                  }
                }
              }
              frame Error {
              }
            }
          }
          event "Refresh Exposure": Value Change {
            w280 = T2 1 items=["FEATURE_FLAG_PRESENCE                 0x00000001", "FEATURE_FLAG_MANUAL                     0x00000002", "FEATURE_FLAG_AUTO                         0x00000004", "FEATURE_FLAG_ONEPUSH                   0x00000008", "FEATURE_FLAG_OFF                            0x00000010", "FEATURE_FLAG_DESC_SUPPORTED    0x00000020", "FEATURE_FLAG_READ_ONLY               0x00000040"] ("uFlags IN")
            w281 = T3 7 items=["FEATURE_BRIGHTNESS", "FEATURE_EXPOSURE", "FEATURE_SHARPNESS", "FEATURE_WHITE_BAL", "FEATURE_HUE", "FEATURE_SATURATION", "FEATURE_GAMMA", "FEATURE_SHUTTER", "FEATURE_GAIN", "FEATURE_IRIS", "FEATURE_FOCUS", "FEATURE_TEMPERATURE", "FEATURE_TRIGGER", "FEATURE_ZOOM", "FEATURE_PAN", "FEATURE_TILT", "FEATURE_OPT_FILTER", "FEATURE_GPIO", "FEATURE_FRAME_RATE", "FEATURE_ROI", "FEATURE_FLIP", "FEATURE_PIXEL_ADDRESSING", "FEATURE_PIXEL_FORMAT", "FEATURE_EXTENDED_SHUTTER", "FEATURE_AUTO_ROI", "FEATURE_LOOKUP_TABLE", "FEATURE_MEMORY_CHANNEL", "FEATURE_WHITE_SHADING", "FEATURE_ROTATE", "FEATURE_IMAGER_CLK_DIVISOR", "FEATURE_TRIG_WITH_CNTRLD_LIGHT", "FEATURE_MAX_PIXEL_SIZE"] ("uFeatureId IN")
            n166 = event-data() -> ()  [unwired: 1 in, 6 out]
            n167 = property on="Camera Handle" class="DigNum (strict)"() -> ("Value"=w277:u32)  [unwired: 2 in, 2 out]
            n168 = property on="Exposure Time" class="Slide (strict)"() -> ("Value"=w279:dbl)  [unwired: 2 in, 2 out]
            n169 = Build Array(w279) -> (w278:dbl[])
            n170 = call <vilib>:"MEPU-CameraFeatures-SetFeature.vi"("hCamera IN"=w277, "uFeatureId IN"=w281, "uFlags IN"=w280, "pParms IN"=w278) -> ()  [unwired: 1 in, 11 out]
          }
          event "Bind Path to Camera": Value Change {
            n171 = event-data() -> ()  [unwired: 1 in, 6 out]
            n172 = property on="Imager" class="Ring (strict)"() -> ("StringsAndValues[]"=w287:T1)  [unwired: 2 in, 2 out]
            n173 = for {
              tunnel: w287 -> [w295] mode=indexing
              tunnel: [w290] -> w286 mode=indexing
              i -> [w291]
              n174 = Unbundle By Name(w295) -> ("String"=w294:string)
              n175 = Concatenate Strings("Choose path to save data\nfrom ", w294) -> (w292:string)
              n176 = Two Button Dialog(message=w292) -> (T button?=w290:bool)  [unwired: 2 in]
              n177 = case shown="True" w290 {
                tunnel: w291 -> [_ w297]
                frame False {
                }
                frame True {
                  n178 = call "File Dialog"() -> ("selected path"=w298:path, "error out"=w296:errorcluster)  [unwired: 12 in, 2 out]
                  n179 = case shown="No Error" w296 {
                    tunnel: w298 -> [w303 _]
                    tunnel: w297 -> [w300 _]
                    frame No Error {
                      n180 = property on="Chemins\n de sauvegarde" class="Arr (strict)"() -> ("Value"=w304:path[])  [unwired: 2 in, 2 out]
                      n181 = Array Size(array=w304) -> (size(s)=w302:i32)
                      n182 = Less Or Equal?(x=w302, y=w300) -> (x <= y?=w301:bool)
                      n183 = case shown="False" w301 {
                        tunnel: w304 -> [w308 w312]
                        tunnel: w303 -> [w306 w310]
                        tunnel: w300 -> [w307 w311]
                        tunnel: [w305 w309] -> w299
                        frame False {
                          n184 = Replace Array Subset(array=w308, new element=w306, index=w307) -> (w305:path[])
                        }
                        frame True {
                          n185 = Insert Into Array(array=w312, index=w311, new element=w310) -> (w309:path[])
                        }
                      }
                      n186 = property on="Chemins\n de sauvegarde" class="Arr (strict)"("Value"=w299) -> ()  [unwired: 2 in, 2 out]
                    }
                    frame Error {
                    }
                  }
                }
              }
            }
            n187 = property on="Imager" class="Ring (strict)"() -> ("Value"=w284:u32)  [unwired: 2 in, 2 out]
            n188 = property on="Imager Serial #" class="Arr (strict)"() -> ("Value"=w283:u32[])  [unwired: 2 in, 2 out]
            n189 = Search 1D Array(1D array=w283, element=w284) -> (index of element=w282:i32)  [unwired: 1 in]
            n190 = Index Array(array=w286, index=w282) -> (element=w285:bool)
            n191 = case shown="True" w285 {
              frame False {
              }
              frame True {
                # "If path to current cam data was changed, update on interface"
                n192 = property on="Chemins\n de sauvegarde" class="Arr (strict)"() -> ("Value"=w289:path[])  [unwired: 2 in, 2 out]
                n193 = Index Array(array=w289) -> (element=w288:path)  [unwired: 1 in]
                n194 = property on="Racine chemin de sauvegarde" class="Path"("Value"=w288) -> ()  [unwired: 2 in, 2 out]
              }
            }
          }
          event "Snap current Data": Value Change {
            n195 = event-data() -> ()  [unwired: 1 in, 6 out]
            n196 = stacked-sequence {
              seq-local: [w320 _] -> [_ w336]
              frame #0 {
                n197 = property on="Racine chemin de sauvegarde" class="Path"() -> ("Value"=w316:path)  [unwired: 2 in, 2 out]
                n198 = property on="Nom du fichier" class="Str"() -> ("Value"=w317:string)  [unwired: 2 in, 2 out]
                n199 = property on="Indice" class="DigNum (strict)"() -> ("Value"=w318:u32)  [unwired: 2 in, 2 out]
                n200 = property on="Overwrite?" class="Bool (strict)"() -> ("Value"=w319:bool)  [unwired: 2 in, 2 out]
                n201 = property on="Automatic\nfolder naming" class="Bool (strict)"() -> ("Value"=w313:bool)  [unwired: 2 in, 2 out]
                n202 = case shown="False" w313 {
                  tunnel: [w323 w334] -> w320
                  tunnel: w319 -> [w324 w333]
                  tunnel: w318 -> [w325 w332]
                  tunnel: w317 -> [w326 w331]
                  tunnel: w316 -> [w327 w330]
                  tunnel: [w322 w329] -> w315
                  tunnel: [w321 w328] -> w314
                  frame False {
                    n203 = call "CheckFolder.vi"("Overwrite?"=w324, "Index"=w325, "File Name"=w326, "Folder Path Control"=w327) -> ("Warning"=w321:bool, "Message"=w322:string, "File Path"=w323:path)  [unwired: 5 in]
                  }
                  frame True {
                    n204 = call "CheckMonthDateFolder.vi"("Overwrite?"=w333, "Index"=w332, "File Name"=w331, "Folder Path Control"=w330) -> ("Warning"=w328:bool, "Message"=w329:string, "File Path"=w334:path)  [unwired: 5 in]
                  }
                }
                n205 = property on="Warning" class="Bool (strict)"("Value"=w314) -> ()  [unwired: 2 in, 2 out]
                n206 = property on="Message" class="Str"("Value"=w315) -> ()  [unwired: 2 in, 2 out]
              }
              frame #1 {
                n207 = Not A Number/Path/Refnum?(number/path/refnum=w336) -> (NaN/Path/Refnum?=w335:bool)
                n208 = case shown="False" w335 {
                  tunnel: w336 -> [w341 _]
                  frame False {
                    # "Save Image\nand data"
                    n209 = property on="Captured Image" class="IntGraph (strict)"() -> ("Value"=w342:dbl[][])  [unwired: 2 in, 2 out]
                    n210 = call "SavePicture.vi"("File Path"=w341, "Image Pixels (U16)"=w342) -> ("error out"=w348:errorcluster)  [unwired: 9 in]
                    n211 = property on="Nom du fichier" class="Str"() -> ("Value"=w340:string)  [unwired: 2 in, 2 out]
                    n212 = property on="Indice" class="DigNum (strict)"() -> ("Value"=w339:u32)  [unwired: 2 in, 2 out]
                    n213 = property on="Exposure Time" class="Slide (strict)"() -> ("Value"=w338:dbl)  [unwired: 2 in, 2 out]
                    n214 = Unbundle By Name(w348) -> ("source"=w345:string, "status"=w346:bool)
                    n215 = call "FindLineAndOverwrite_Double.vi"("Exposure path"=w341, "Name"=w340, "Index"=w339, "Exposure"=w338) -> ("error out"=w337:errorcluster)  [unwired: 11 in]
                    n216 = Unbundle By Name(w337) -> ("status"=w347:bool, "source"=w349:string)
                    n217 = Or(x=w346, y=w347) -> (x .or. y?=w344:bool)
                    n218 = case shown="False" w344 {
                      tunnel: w349 -> [_ w353]
                      tunnel: w345 -> [_ w356]
                      tunnel: "\r\n" -> [_ w354]
                      frame False {
                        n219 = property on="Mode de Sauvegarde" class="Ring (strict)"() -> ("Value"=w351:u16)  [unwired: 2 in, 2 out]
                        n220 = property on="Indice" class="DigNum (strict)"() -> ("Value"=w352:u32)  [unwired: 2 in, 2 out]
                        n221 = Add(x=w352, y=w351) -> (x+y=w350:u32)
                        n222 = property on="Indice" class="DigNum (strict)"("Value"=w350) -> ()  [unwired: 2 in, 2 out]
                      }
                      frame True {
                        n223 = Concatenate Strings(w356, w354, w353) -> (w355:string)
                        n224 = property on="Message" class="Str"("Value"=w355) -> ()  [unwired: 2 in, 2 out]
                      }
                    }
                  }
                  frame True {
                  }
                }
              }
            }
          }
        }
      }
      n225 = property on="Error OUT" class="Clust (strict)"("Value"=w45) -> ()  [unwired: 2 in, 2 out]
    }
    frame #4 {
      w358 = T4 2 items=["START_STREAM", "PAUSE_STREAM", "STOP_STREAM"] ("uStreamState IN")
      # "Ignore errors here to ensure as\ncomplete a clean up as possible."
      n226 = property on="Camera Handle" class="DigNum (strict)"() -> ("Value"=w357:u32)  [unwired: 2 in, 2 out]
      n227 = call <vilib>:"MEPU-Acquisition-SetStreamState.vi"("hCamera IN"=w357, "uStreamState IN"=w358) -> ("hCamera OUT"=w360:u32)  [unwired: 12 in, 1 out]
      n228 = call <vilib>:"MEPU-Initialization-Uninitialize.vi"("hCamera IN"=w360) -> ("Error OUT"=w359:errorcluster)  [unwired: 14 in]
      n229 = stacked-sequence {
        tunnel: w359 -> [_]
        frame #0 {
          n230 = call <vilib>:"MEPU-Initialization-UninitializeSystem.vi"() -> ()  [unwired: 15 in, 1 out]
        }
      }
    }
  }
